vi "Fetch.vi"(8 "error in (no error)":errorcluster, 9 "Timeout (10000 ms)":u32=10000, 11 "VISA resource name":refnum<visa-resource-name>) -> (0 "error out":errorcluster, 2 "Measurements":dbl[](array[numeric]), 3 "VISA resource name out":refnum<visa-resource-name>)   [LabVIEW 2014, in "Fluke 884X Series.lvlib"]
doc: "Fetches the measurement according to the instrument model, trigger source, and math configuration.\n\n<B>Note:</B>\n\nThis VI does not check the instrument status. Typically, you call this VI only in a sequence of calls to other low-level instrument driver VIs. The sequence performs one operation. You use the low-level VIs to optimize one or more aspects of interaction with the instrument. If you want to check the instrument status, call the <B>Error Query VI</B> at the conclusion of the sequence."
uses:
  Fluke 884X Series.lvlib
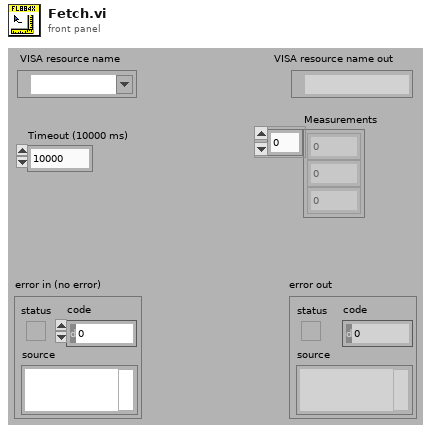
[diagram p1: front panel]
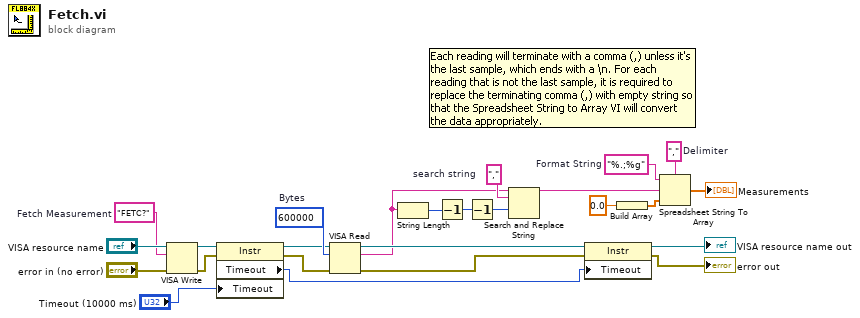
[diagram p0: block diagram]
diagram:
  w6 = ","  # search string
  w7 = "FETC?"  # Fetch Measurement
  w17 = ","  # Delimiter
  w18 = "%.;%g"  # Format String
  w21 = u32 600000  # Bytes
  n1 = VISA Write(VISA resource name="VISA resource name", write buffer=w7, error in (no error)="error in (no error)") -> (VISA resource name out=w11:refnum<visa-resource-name>, error out=w25:errorcluster)  [unwired: 1 out]
  n2 = property class="Instr"(reference=w11, error in=w25, "Timeout"="Timeout (10000 ms)") -> (reference out=w10:refnum<visa-resource-name>, error out=w22:errorcluster, "Timeout"=w15:u32)
  n3 = VISA Read(VISA resource name=w10, byte count=w21, error in (no error)=w22) -> (VISA resource name out=w9:refnum<visa-resource-name>, read buffer=w1:string, error out=w16:errorcluster)  [unwired: 1 out]
  n4 = String Length(string=w1) -> (length=w3:i32)
  n5 = Decrement(x=w3) -> (x-1=w4:i32)
  n6 = Decrement(x=w4) -> (x-1=w5:i32)
  n7 = Search and Replace String(input string=w1, search string=w6, offset=w5) -> (result string=w2:string)  [unwired: 5 in, 3 out]
  n8 = property class="Instr"(reference=w9, error in=w16, "Timeout"=w15) -> (reference out=→"VISA resource name out":refnum<visa-resource-name>, error out=→"error out":errorcluster)
  n9 = Build Array(0.0 ("element")) -> (w19:dbl[])
  n10 = Spreadsheet String To Array(delimiter (Tab)=w17, format string=w18, spreadsheet string=w2, array type (2D Dbl)=w19) -> (array=→"Measurements":dbl[])
